vi "GetInheritance.vi"(0 "ClassReaderNative in":refnum<class "ClassReaderNative.lvclass">, 5 "error in (no error)":errorcluster) -> (14 "ClassReaderNative out":refnum<class "ClassReaderNative.lvclass">, 15 "Inheritance":path[](array[path]), 16 "Inherits":bool, 19 "error out":errorcluster)   [LabVIEW 2014, in "ClassReaderNative.lvclass"]
uses:
  <resource>/Framework/Providers/Open_GDS/ClassProviders/Provider_LvNativeClass/ClassReaderNative_class/ClassReaderNative.lvclass
  <resource>/Framework/Providers/Open_GDS/ClassProviders/Provider_LvNativeClass/ClassReaderNative_class/ClassReaderNative.lvclass/ClassReaderNative.ctl
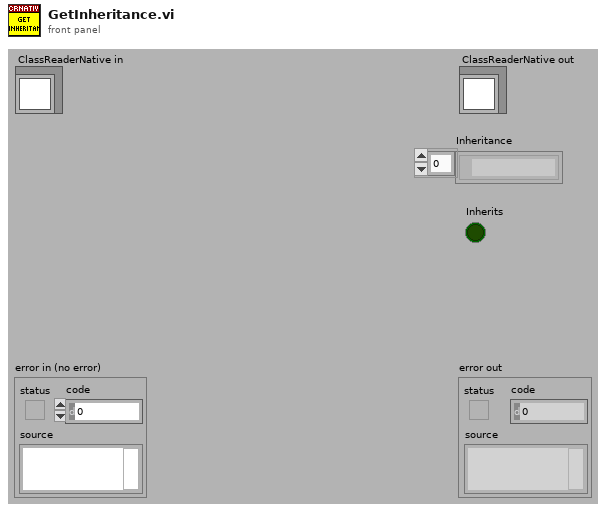
[diagram p1: front panel]
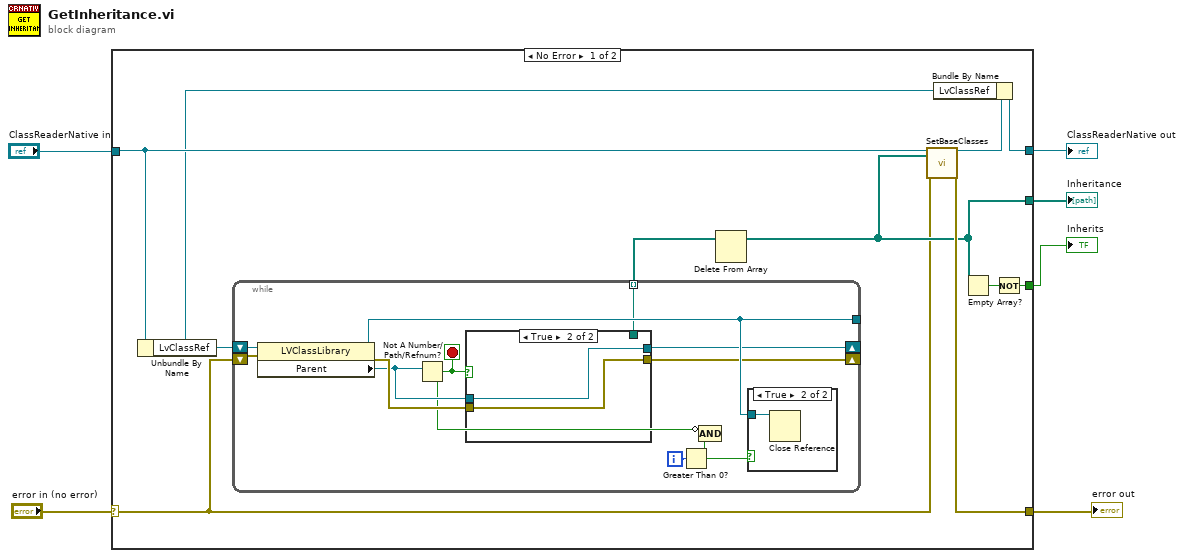
[diagram p0: block diagram]
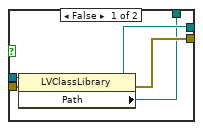
[diagram p2: hidden frame]
diagram:
  n1 = case shown="No Error" "error in (no error)" {
    selector: "error in (no error)" -> [w7 w37]
    tunnel: [w12 _] -> w6
    tunnel: [w14 _] -> w5
    tunnel: "ClassReaderNative in" -> [w9 w36]
    tunnel: [w13 w37] -> w2
    tunnel: [w10 w36] -> w1
    frame No Error {
      n2 = Unbundle By Name(w9) -> ("LvClassRef"=w8:refnum<vi>)
      n3 = while {
        shift-right: [w23] -> _
        shift-left: w8 -> [w27]
        tunnel: [w25] -> _
        shift-right: [w21] -> _
        shift-left: w7 -> [w26]
        tunnel: [w20] -> w15 mode=indexing
        i -> [w24]
        stop <- w18 stop-if-true
        n4 = property class="LVClassLibrary"(reference=w27, error in=w26) -> (reference out=w25:refnum<vi>, error out=w22:errorcluster, "Parent"=w19:refnum<vi>)
        n5 = Not A Number/Path/Refnum?(number/path/refnum=w19) -> (NaN/Path/Refnum?=w18:bool)
        n6 = case shown="True" w18 {
          tunnel: [w32 w33] -> w23
          tunnel: w22 -> [w31 w34]
          tunnel: [w30 w34] -> w21
          tunnel: [w29 _] -> w20
          tunnel: w19 -> [w28 w33]
          frame False {
            n7 = property class="LVClassLibrary"(reference=w28, error in=w31) -> (reference out=w32:refnum<vi>, error out=w30:errorcluster, "Path"=w29:path)
          }
          frame True {
          }
        }
        n8 = Greater Than 0?(x=w24) -> (x > 0?=w17:bool)
        n9 = Compound Arithmetic op=AND(invert w18, w17) -> ()  [unwired: 1 out]
        n10 = case shown="True" w17 {
          tunnel: w25 -> [_ w35]
          frame False {
          }
          frame True {
            n11 = Close Reference(reference=w35) -> ()  [unwired: 1 in, 1 out]
          }
        }
      }
      n12 = Delete From Array(array=w15) -> (array with subset deleted=w12:path[])  [unwired: 2 in, 1 out]
      n13 = call-dynamic "SetBaseClasses.vi"("ClassReader in"=w9, "Inheritance"=w12, "error in (no error)"=w7) -> ("ClassReader out"=w11:refnum<class "ClassReaderNative.lvclass">, "error out"=w13:errorcluster)  [unwired: 15 in]
      n14 = Bundle By Name(cluster=w11, "LvClassRef"=w8) -> (w10:refnum<class "ClassReaderNative.lvclass">)
      n15 = Empty Array?(array=w12) -> (empty?=w16:bool)
      n16 = Not(x=w16) -> (.not. x?=w14:bool)
    }
    frame Error {
    }
  }
  "ClassReaderNative out" <- w1
  "Inheritance" <- w6
  "Inherits" <- w5
  "error out" <- w2
